vi "TESTnew-PI.vi"() -> ()   [LabVIEW 2014]
panel:
  in  "Rec. table":i32
  in  "Value":string[](array[string])
  in  "Trigger source":i32[](array[numeric])
  in  "DataRecorderTable":i32[](array[numeric])
  in  "Rec. table IDs":i32[](array[numeric])
  in  "Nmax":i32=1024
  in  "N":i32=100
  out "Data":dbl[][](array[numeric]) format="%.6f"
  out "Names":string[](array[string])
  out "Waveform Graph":dbl[](graph)
  in  "Source ID":string
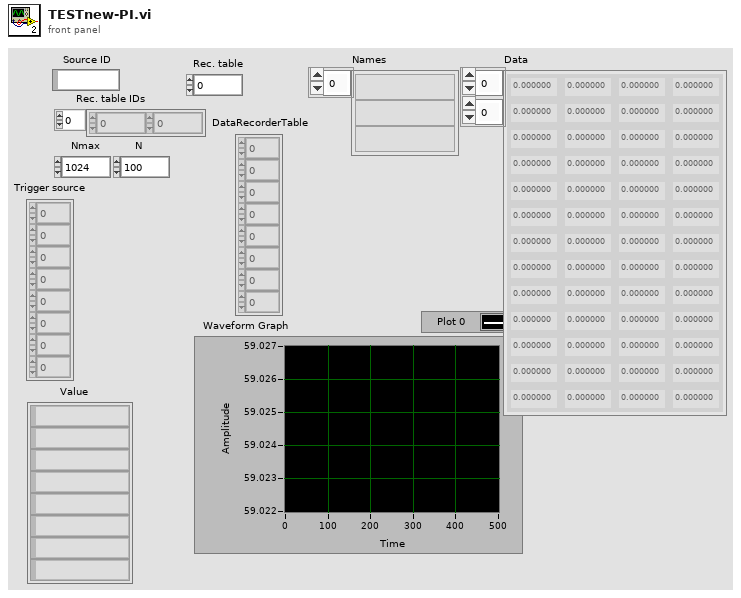
[diagram p1: front panel]
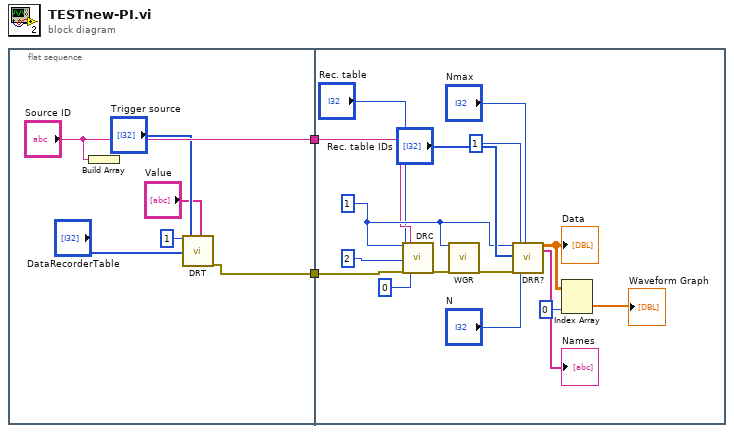
[diagram p0: block diagram]
diagram:
  n1 = flat-sequence {
    tunnel: ["Source ID"] -> w2
    tunnel: [w3] -> w1
    tunnel: w2 -> [w11]
    tunnel: w1 -> [w10]
    frame #0 {
      n2 = Build Array("Source ID") -> ()  [unwired: 1 out]
      n3 = call "DRT.vi"("System no."=1, "DataRecorderTable"="DataRecorderTable", "Trigger source"="Trigger source", "Value"="Value") -> ("error out"=w3:errorcluster)  [unwired: 1 in, 14 out]
    }
    frame #1 {
      w12 = 1 ("System no.")
      n4 = call "DRC.vi"("System no."=w12, "Rec. table"="Rec. table", "Rec. option"=2, "error in"=w10, "Source ID"=w11, "Trigger option"=0) -> ("error out"=w24:errorcluster)  [unwired: 13 out]
      n5 = call "WGR.vi"("System no."=w12, "error in"=w24) -> ("error out"=w23:errorcluster)  [unwired: 2 in, 15 out]
      n6 = call "DRR?.vi"("System no."=w12, "Rec. table IDs"="Rec. table IDs", "error in"=w23, "Xo"=1, "N"="N", "Nmax"="Nmax") -> ("Data"=w17:dbl[][], "Names"=→"Names":string[])  [unwired: 2 in, 10 out]
      "Data" <- w17
      n7 = Index Array(array=w17, index (col)=0 ("disabled index (col)")) -> (element=→"Waveform Graph":dbl[])  [unwired: 1 in]
    }
  }
